vi "Brushless Speed Calc (RT).vi"(7 "Data In":dbl[](array[numeric])) -> (8 "Speed":dbl)   [LabVIEW 2013]
panel:
  out "Waveform Chart":dbl(graph)
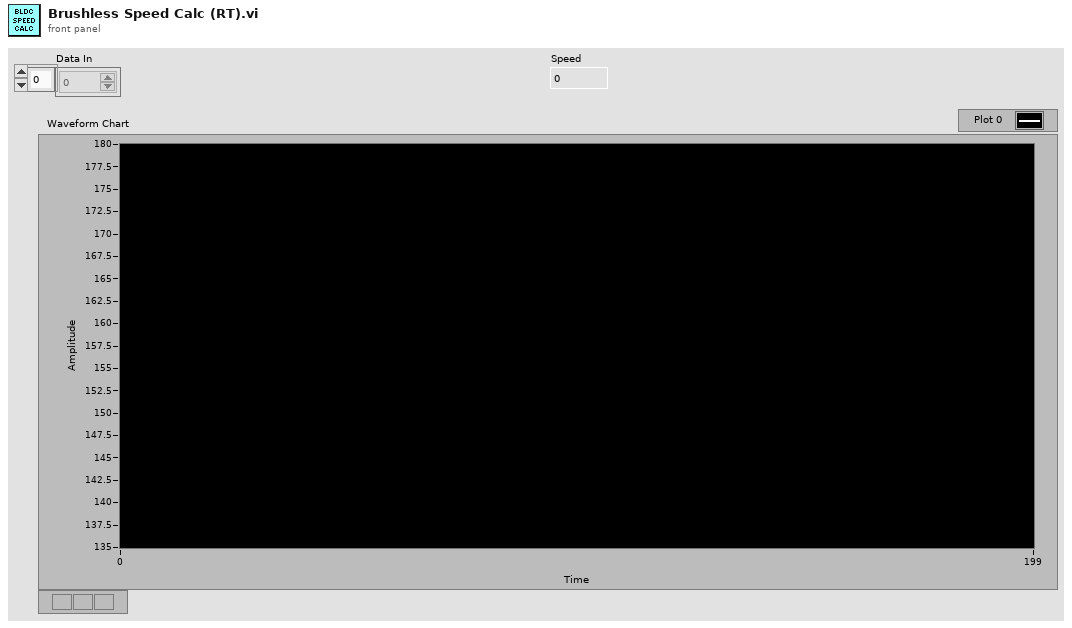
[diagram p1: front panel]
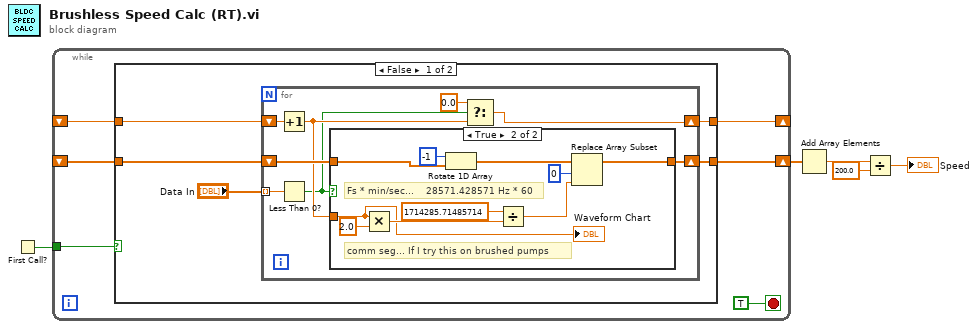
[diagram p0: block diagram]
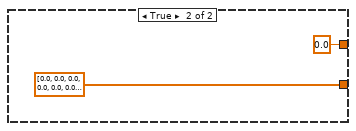
[diagram p3: hidden frame]
diagram:
  n1 = First Call?() -> (First Call?: T/F=w5:bool)
  n2 = while {
    tunnel: w5 -> [w10]
    shift-right: [w9] -> w1
    shift-left: _ -> [w8]
    shift-right: [w7] -> _
    shift-left: _ -> [w6]
    stop <- TRUE stop-if-true
    n3 = case shown="False" w10 {
      tunnel: [w15 dbl[] [0.0, 0.0, 0.0, 0.0, 0.0, 0.0, 0.0, 0.0, 0.0, 0.0, 0.0, 0.0, 0.0, 0.0, 0.0, 0.0, 0.0, 0.0, 0.0, 0.0, 0.0, 0.0, 0.0, 0.0, 0.0, 0.0, 0.0, 0.0, 0.0, 0.0, 0.0, 0.0, 0.0, 0.0, 0.0, 0.0, 0.0, 0.0, 0.0, 0.0, 0.0, 0.0, 0.0, 0.0, 0.0, 0.0, 0.0, 0.0, 0.0, 0.0, 0.0, 0.0, 0.0, 0.0, 0.0, 0.0, 0.0, 0.0, 0.0, 0.0, 0.0, 0.0, 0.0, 0.0, 0.0, 0.0, 0.0, 0.0, 0.0, 0.0, 0.0, 0.0, 0.0, 0.0, 0.0, 0.0, 0.0, 0.0, 0.0, 0.0, 0.0, 0.0, 0.0, 0.0, 0.0, 0.0, 0.0, 0.0, 0.0, 0.0, 0.0, 0.0, 0.0, 0.0, 0.0, 0.0, 0.0, 0.0, 0.0, 0.0, 0.0, 0.0, 0.0, 0.0, 0.0, 0.0, 0.0, 0.0, 0.0, 0.0, 0.0, 0.0, 0.0, 0.0, 0.0, 0.0, 0.0, 0.0, 0.0, 0.0, 0.0, 0.0, 0.0, 0.0, 0.0, 0.0, 0.0, 0.0, 0.0, 0.0, 0.0, 0.0, 0.0, 0.0, 0.0, 0.0, 0.0, 0.0, 0.0, 0.0, 0.0, 0.0, 0.0, 0.0, 0.0, 0.0, 0.0, 0.0, 0.0, 0.0, 0.0, 0.0, 0.0, 0.0, 0.0, 0.0, 0.0, 0.0, 0.0, 0.0, 0.0, 0.0, 0.0, 0.0, 0.0, 0.0, 0.0, 0.0, 0.0, 0.0, 0.0, 0.0, 0.0, 0.0, 0.0, 0.0, 0.0, 0.0, 0.0, 0.0, 0.0, 0.0, 0.0, 0.0, 0.0, 0.0, 0.0, 0.0, 0.0, 0.0, 0.0, 0.0, 0.0, 0.0, 0.0, 0.0, 0.0, 0.0, 0.0, 0.0]] -> w9
      tunnel: w8 -> [w16 _]
      tunnel: [w14 0.0 ("t")] -> w7
      tunnel: w6 -> [w13 _]
      frame False {
        n4 = for {
          tunnel: "Data In" -> [w18] mode=indexing
          shift-right: [w23] -> w14
          shift-left: w13 -> [w24]
          shift-right: [w20] -> w15
          shift-left: w16 -> [w21]
          n5 = Increment(x=w24) -> (x+1=w19:dbl)
          n6 = Less Than 0?(x=w18) -> (x < 0?=w17:bool)
          n7 = case shown="True" w17 {
            tunnel: w21 -> [w25 w35]
            tunnel: [w25 w32] -> w20
            tunnel: w19 -> [_ w26]
            frame False {
            }
            frame True {
              # "comm seg... If I try this on brushed pumps"
              # "Fs * min/sec...    28571.428571 Hz * 60"
              n8 = Multiply(x=w26, y=2.0) -> (x*y=w29:dbl)
              n9 = Rotate 1D Array(1:w35, 2:-1 ("n")) -> (0:w33:dbl[])
              n10 = Divide(x=1714285.71485714, y=w29) -> (x/y=w28:dbl)
              n11 = Replace Array Subset(array=w33, new element=w28, index=0) -> (w32:dbl[])
              "Waveform Chart" <- w26
            }
          }
          n12 = Select(t=0.0, s=w17, f=w19) -> (s? t:f=w23:dbl)
        }
      }
      frame True {
      }
    }
  }
  n13 = Add Array Elements(numeric array=w1) -> (sum=w3:dbl)
  n14 = Divide(x=w3, y=200.0) -> (x/y=→"Speed":dbl)
